vi "ProgramControlFault.vi"(0 "Front Panel Controls in":T1) -> (14 "Front Panel Controls out":T1)   [LabVIEW 2019, in "Universal Robot.lvclass"]
uses:
  Universal Robot.lvclass
  ProgramControlFPControls.ctl
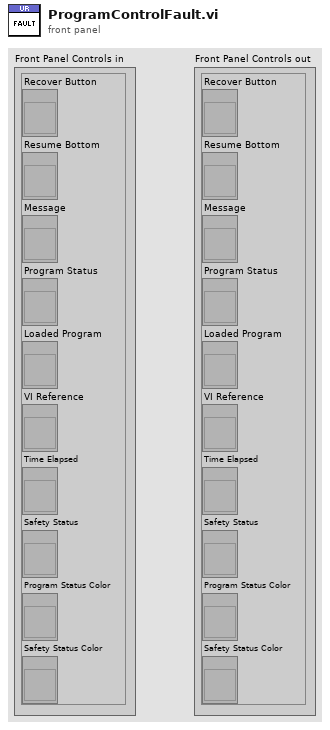
[diagram p1: front panel]
types:
  T1 = typedef "Universal Robot.lvclass/ProgramControlFPControls.ctl" = cluster{"Recover Button":refnum<vi>, "Resume Bottom":refnum<vi>, "Message":refnum<vi>, "Program Status":refnum<vi>, "Loaded Program":refnum<vi>, "VI Reference":refnum<vi>, "Time Elapsed":refnum<vi>, "Safety Status":refnum<vi>, "Program Status Color":refnum<vi>, "Safety Status Color":refnum<vi>}
  T2 = enum8{"Enabled", "Disabled", "Disabled and Grayed Out"}
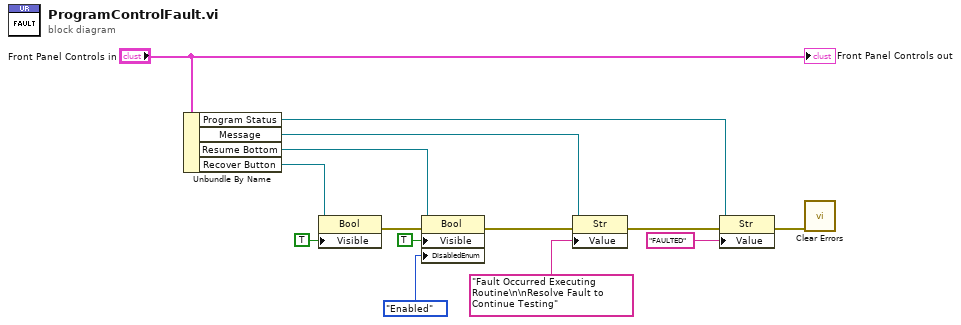
[diagram p0: block diagram]
diagram:
  n1 = Unbundle By Name("Front Panel Controls in") -> ("Program Status"=w4:refnum<vi>, "Message"=w8:refnum<vi>, "Resume Bottom"=w10:refnum<vi>, "Recover Button"=w13:refnum<vi>)
  n2 = property class="Bool"(reference=w13, "Visible"=TRUE) -> (error out=w11:errorcluster)  [unwired: 1 in, 1 out]
  n3 = property class="Bool"(reference=w10, error in=w11, "Visible"=TRUE, "DisabledEnum"=T2."Enabled" ("Disabled")) -> (error out=w7:errorcluster)  [unwired: 1 out]
  n4 = property class="Str"(reference=w8, error in=w7, "Value"="Fault Occurred Executing Routine\n\nResolve Fault to Continue Testing") -> (error out=w5:errorcluster)  [unwired: 1 out]
  n5 = property class="Str"(reference=w4, error in=w5, "Value"="FAULTED") -> (error out=w2:errorcluster)  [unwired: 1 out]
  n6 = call <vilib>:"Clear Errors.vi"("error in (no error)"=w2) -> ()  [unwired: 5 in, 2 out]
  "Front Panel Controls out" <- "Front Panel Controls in"
